vi "Update Counters.vi"(7 "Current Missing Points":i32, 8 "Current Duplicated Points":i32, 9 "Producer Iterations":i32, 10 "Previous Producer Iterations":i32) -> (0 "Updated Missing Points":i32, 1 "Updated Duplicated Points":i32)   [LabVIEW 2012]
doc: "This VI uses the current and previous producer loop iteration count to determine if the consumer loop is missing data or duplicating data. Depending on if data is missing or duplicated, this VI updates the missing or duplicated count."
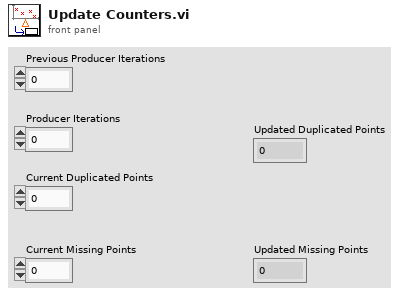
[diagram p1: front panel]
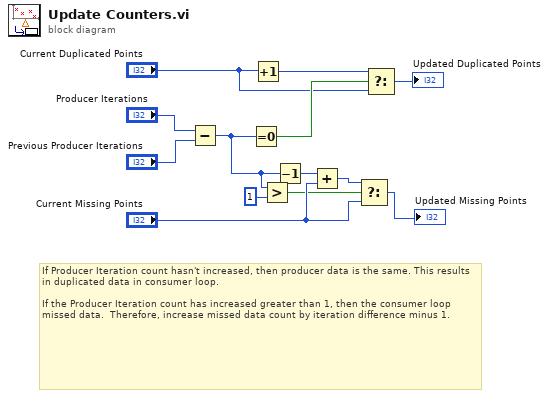
[diagram p0: block diagram]
diagram:
  # "If Producer Iteration count hasn't increased, then producer data is the same. This results in duplicated data in consumer loop.\n\nIf the Producer Iteration count has increased greater than 1, then the consumer loop missed data.  Therefore, increase missed data count by iteration difference minus 1."
  n1 = Subtract(x="Producer Iterations", y="Previous Producer Iterations") -> (x-y=w6:i32)
  n2 = Equal To 0?(x=w6) -> (x = 0?=w9:bool)
  n3 = Increment(x="Current Duplicated Points") -> (x+1=w8:i32)
  n4 = Greater?(x=w6, y=1) -> (0:w3:bool)
  n5 = Decrement(x=w6) -> (x-1=w1:i32)
  n6 = Add(x=w1, y="Current Missing Points") -> (x+y=w5:i32)
  n7 = Select(t=w5, s=w3, f="Current Missing Points") -> (s? t:f=→"Updated Missing Points":i32)
  n8 = Select(t=w8, s=w9, f="Current Duplicated Points") -> (s? t:f=→"Updated Duplicated Points":i32)
